vi "myfirst3.vi"() -> ()   [LabVIEW 2020]
panel:
  out "Boolean 3":bool
  out "Boolean 2":bool
  in  "stop":bool
  in  "Boolean":bool
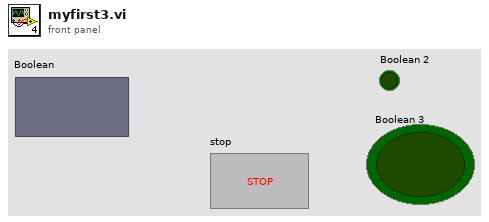
[diagram p1: front panel]
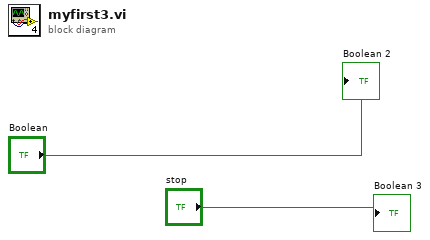
[diagram p0: block diagram]
diagram:
  "Boolean 2" <- "Boolean"
  "Boolean 3" <- "stop"
